vi "log analysis_gps.vi"() -> ()   [LabVIEW 2018] (continued)
0*55731318\n\t", "DUALANTENNAHEADINGA,USB3,0,53.5,FINESTEERING,2107,283868.900,02000000,d426,15824;INSUFFICIENT_OBS,NONE,-1.000000000,0.000000000,0.000000000,0.0,0.000000000,0.000000000,\"631T\",14,3,3,3,04,00,20,00*2bda417b\n\t", "INSPVAXA,USB3,0,47.5,FINESTEERING,2107,283869.400,02000000,471d,15824;INS_ALIGNMENT_COMPLETE,INS_RTKFIXED,37.37070477498,126.72137878954,8.8182,22.3000,-0.3794,-0.2856,0.0387,-0.580248712,0.693765436,214.050059591,0.4343,0.3016,0.5953,0.1139,0.0951,0.0843,0.0965,0.1004,5.1447,0f000001,0*5005ba7a\n\t", "INSPVAXA,USB3,0,47.5,FINESTEERING,2107,283869.900,02000000,471d,15824;INS_ALIGNMENT_COMPLETE,INS_RTKFIXED,37.37070349907,126.72137747347,8.8234,22.3000,-0.3765,-0.2687,0.0325,-0.595922163,0.823980271,213.804726387,0.4343,0.3016,0.5953,0.1139,0.0951,0.0843,0.0965,0.1004,5.1447,0f000001,0*b08e18e5\n\t", "INSPVAXA,USB3,0,48.0,FINESTEERING,2107,283870.400,02000000,471d,15824;INS_ALIGNMENT_COMPLETE,INS_RTKFIXED,37.37070163427,126.72137570159,8.8300,22.3000,-0.3041,-0.2407,0.0180,-0.604642888,0.778196285,214.030795943,0.4340,0.3016,0.5956,0.1141,0.0959,0.0845,0.0966,0.1004,5.1433,0f000001,0*cb822ea1\n\t", "INSPVAXA,USB3,0,48.0,FINESTEERING,2107,283870.900,02000000,471d,15824;INS_ALIGNMENT_COMPLETE,INS_RTKFIXED,37.37069994386,126.72137408130,8.8327,22.3000,-0.4129,-0.3185,0.0299,-0.561714396,1.101086671,213.985768500,0.4340,0.3016,0.5956,0.1141,0.0959,0.0845,0.0966,0.1004,5.1433,0f000001,0*097c1e24\n\t", "INSPVAXA,USB3,0,50.0,FINESTEERING,2107,283871.400,02000000,471d,15824;INS_ALIGNMENT_COMPLETE,INS_RTKFIXED,37.37069831939,126.72137250494,8.8386,22.3000,-0.3879,-0.3050,0.0340,-0.603840717,0.986135442,213.822522610,0.4341,0.3014,0.5961,0.1146,0.0956,0.0852,0.0966,0.1005,5.1404,0f000001,0*99650335\n\t", "INSPVAXA,USB3,0,50.0,FINESTEERING,2107,283871.900,02000000,471d,15824;INS_ALIGNMENT_COMPLETE,INS_RTKFIXED,37.37069663076,126.72137084332,8.8454,22.3000,-0.3570,-0.2814,0.0330,-0.426296070,0.946461964,213.763011209,0.4341,0.3014,0.5961,0.1146,0.0956,0.0852,0.0966,0.1005,5.1404,0f000001,0*8cc6f2c5\n\t", "INSPVAXA,USB3,0,48.5,FINESTEERING,2107,283872.400,02000000,471d,15824;INS_ALIGNMENT_COMPLETE,INS_RTKFIXED,37.37069491831,126.72136922755,8.8525,22.3000,-0.3761,-0.2771,0.0323,-0.638578544,0.908546721,213.728365329,0.4343,0.3024,0.5968,0.1148,0.0958,0.0857,0.0966,0.1006,5.1403,0f000001,0*b6cc0c4e\n\t", "INSPVAXA,USB3,0,48.5,FINESTEERING,2107,283872.900,02000000,471d,15824;INS_ALIGNMENT_COMPLETE,INS_RTKFIXED,37.37069321684,126.72136760945,8.8593,22.3000,-0.3790,-0.2963,0.0419,-0.436104629,0.871418994,213.562317886,0.4343,0.3024,0.5968,0.1148,0.0958,0.0857,0.0966,0.1006,5.1403,0f000001,0*c4a88a6a\n\t", "INSPVAXA,USB3,0,49.5,FINESTEERING,2107,283873.400,02008000,471d,15824;INS_ALIGNMENT_COMPLETE,INS_RTKFIXED,37.37069152716,126.72136602353,8.8633,22.3000,-0.3871,-0.2959,0.0071,-0.372350545,0.744743761,213.502289859,0.4348,0.3034,0.5975,0.1151,0.0961,0.0863,0.0967,0.1006,5.1413,0f000001,0*db4d8b18\n\t", "INSPVAXA,USB3,0,49.5,FINESTEERING,2107,283873.900,02008000,471d,15824;INS_ALIGNMENT_COMPLETE,INS_RTKFIXED,37.37068980188,126.72136442451,8.8669,22.3000,-0.3821,-0.2876,0.0223,-0.542252908,0.493927279,213.372683943,0.4348,0.3034,0.5975,0.1151,0.0961,0.0863,0.0967,0.1006,5.1413,0f000001,0*34acffbe\n\t", "INSPVAXA,USB3,0,52.5,FINESTEERING,2107,283874.400,02008000,471d,15824;INS_ALIGNMENT_COMPLETE,INS_RTKFIXED,37.37068808694,126.72136282059,8.8713,22.3000,-0.3710,-0.2644,0.0357,-0.579423021,0.489216985,213.355766858,0.4351,0.3041,0.5984,0.1155,0.0964,0.0870,0.0968,0.1007,5.1427,0f000001,0*1b568777\n\t", "DUALANTENNAHEADINGA,USB3,0,52.5,FINESTEERING,2107,283874.900,02008000,d426,15824;INSUFFICIENT_OBS,NONE,-1.000000000,0.000000000,0.000000000,0.0,0.000000000,0.000000000,\"631T\",11,3,3,3,04,00,20,00*2cd613df\n\t", "INSPVAXA,USB3,0,49.5,FINESTEERING,2107,283875.400,02008000,471d,15824;INS_ALIGNMENT_COMPLETE,INS_RTKFIXED,37.37068468930,126.72135963115,8.8825,22.3000,-0.3622,-0.2842,0.0299,-0.576500581,0.429092334,213.280984070,0.4354,0.3044,0.5994,0.1156,0.0965,0.0875,0.0969,0.1007,5.1441,0f000001,0*e8de9d75\n\t", "INSPVAXA,USB3,0,49.5,FINESTEERING,2107,283875.900,02008000,471d,15824;INS_ALIGNMENT_COMPLETE,INS_RTKFIXED,37.37068297802,126.72135803904,8.8854,22.3000,-0.3707,-0.2810,0.0365,-0.547997166,0.698496112,213.263606551,0.4354,0.3044,0.5994,0.1156,0.0965,0.0875,0.0969,0.1007,5.1441,0f000001,0*65e2a656\n\t", "INSPVAXA,USB3,0,44.0,FINESTEERING,2107,283876.400,02008000,471d,15824;INS_ALIGNMENT_COMPLETE,INS_RTKFIXED,37.37068125444,126.72135642974,8.8888,22.3000,-0.3786,-0.2878,0.0233,-0.531966030,0.387673420,213.289464944,0.4359,0.3047,0.6005,0.1161,0.0970,0.0885,0.0969,0.1008,5.1456,0f000001,0*b4409e90\n\t", "INSPVAXA,USB3,0,44.0,FINESTEERING,2107,283876.900,02008000,471d,15824;INS_ALIGNMENT_COMPLETE,INS_RTKFIXED,37.37067957761,126.72135484740,8.8937,22.3000,-0.4026,-0.3012,0.0273,-0.420783044,0.494040879,213.316912941,0.4359,0.3047,0.6005,0.1161,0.0970,0.0885,0.0969,0.1008,5.1456,0f000001,0*00e3c1db\n\t", "DUALANTENNAHEADINGA,USB3,0,43.5,FINESTEERING,2107,283877.400,02000000,d426,15824;INSUFFICIENT_OBS,NONE,-1.000000000,0.000000000,0.000000000,0.0,0.000000000,0.000000000,\"631T\",12,3,3,3,04,00,20,00*231fd75a\n\t", "INSPVAXA,USB3,0,43.5,FINESTEERING,2107,283877.900,02000000,471d,15824;INS_ALIGNMENT_COMPLETE,INS_RTKFIXED,37.37067617157,126.72135158509,8.9007,22.3000,-0.3585,-0.2879,0.0250,-0.387485023,0.488203983,213.381189141,0.4358,0.3051,0.6016,0.1150,0.0957,0.0873,0.0971,0.1009,5.1472,0f000001,0*c9483ecc\n\t", "DUALANTENNAHEADINGA,USB3,0,49.5,FINESTEERING,2107,283878.400,02000000,d426,15824;INSUFFICIENT_OBS,NONE,-1.000000000,0.000000000,0.000000000,0.0,0.000000000,0.000000000,\"631T\",9,3,3,3,04,00,20,00*27e46637\n\t", "INSPVAXA,USB3,0,49.5,FINESTEERING,2107,283878.900,02000000,471d,15824;INS_ALIGNMENT_COMPLETE,INS_RTKFIXED,37.37067289269,126.72134842166,8.9107,22.3000,-0.2321,-0.2053,0.0305,-0.361897679,0.347183543,213.363814143,0.4356,0.3048,0.6022,0.1141,0.0948,0.0861,0.0972,0.1010,5.1487,0f000001,0*7c1228c2\n\t", "INSPVAXA,USB3,0,50.0,FINESTEERING,2107,283879.400,02000000,471d,15824;INS_ALIGNMENT_COMPLETE,INS_RTKFIXED,37.37067136914,126.72134696073,8.9138,22.3000,-0.4356,-0.3421,0.0457,-0.368595541,0.477690460,213.236251513,0.4352,0.3048,0.6024,0.1137,0.0954,0.0849,0.0973,0.1011,5.1500,0f000001,0*de91db37\n\t", "DUALANTENNAHEADINGA,USB3,0,50.0,FINESTEERING,2107,283879.900,02000000,d426,15824;INSUFFICIENT_OBS,NONE,-1.000000000,0.000000000,0.000000000,0.0,0.000000000,0.000000000,\"631T\",11,3,3,3,04,00,20,00*7e5de74c\n\t", "INSPVAXA,USB3,0,53.0,FINESTEERING,2107,283880.400,02000000,471d,15824;INS_ALIGNMENT_COMPLETE,INS_RTKFIXED,37.37066797060,126.72134375029,8.9215,22.3000,-0.3538,-0.2783,0.0388,-0.597615608,0.513014169,213.355161065,0.4357,0.3062,0.6023,0.1133,0.0940,0.0839,0.0973,0.1012,5.1494,0f000001,0*cddeff4e\n\t", "INSPVAXA,USB3,0,53.0,FINESTEERING,2107,283880.900,02000000,471d,15824;INS_ALIGNMENT_COMPLETE,INS_RTKFIXED,37.37066635165,126.72134221442,8.9278,22.3000,-0.3658,-0.2852,0.0396,-0.626245150,0.597396810,213.371902809,0.4357,0.3062,0.6023,0.1133,0.0940,0.0839,0.0973,0.1012,5.1494,0f000001,0*bdd5d949\n\t", "DUALANTENNAHEADINGA,USB3,0,50.5,FINESTEERING,2107,283881.400,02000000,d426,15824;INSUFFICIENT_OBS,NONE,-1.000000000,0.000000000,0.000000000,0.0,0.000000000,0.000000000,\"631T\",11,3,3,3,04,00,20,00*4d958a84\n\t", "INSPVAXA,USB3,0,50.5,FINESTEERING,2107,283881.900,02000000,471d,15824;INS_ALIGNMENT_COMPLETE,INS_RTKFIXED,37.37066299197,126.72133897955,8.9361,22.3000,-0.3474,-0.2868,0.0393,-0.593672744,0.610910921,213.511371032,0.4358,0.3048,0.6020,0.1139,0.0948,0.0841,0.0973,0.1012,5.1504,0f000001,0*060d8030\n\t", "DUALANTENNAHEADINGA,USB3,0,51.5,FINESTEERING,2107,283882.400,02000000,d426,15824;INSUFFICIENT_OBS,NONE,-1.000000000,0.000000000,0.000000000,0.0,0.000000000,0.000000000,\"631T\",12,3,3,3,04,00,20,00*3cefd7e2\n\t", "INSPVAXA,USB3,0,51.5,FINESTEERING,2107,283882.900,02000000,471d,15824;INS_ALIGNMENT_COMPLETE,INS_RTKFIXED,37.37065963052,126.72133572900,8.9416,22.3000,-0.3499,-0.2875,0.0236,-0.546470396,0.861326947,213.517075808,0.4357,0.3040,0.6014,0.1142,0.0952,0.0840,0.0973,0.1012,5.1519,0f000001,0*24ce4552\n\t", "INSPVAXA,USB3,0,52.0,FINESTEERING,2107,283883.400,02000000,471d,15824;INS_ALIGNMENT_COMPLETE,INS_RTKFIXED,37.37065796164,126.72133411405,8.9451,22.3000,-0.3685,-0.2983,0.0398,-0.521036438,0.724479041,213.604247881,0.4353,0.3043,0.6007,0.1142,0.0953,0.0836,0.0972,0.1012,5.1533,0f000001,0*63d3ff51\n\t", "DUALANTENNAHEADINGA,USB3,0,52.0,FINESTEERING,2107,283883.900,02000000,d426,15824;INSUFFICIENT_OBS,NONE,-1.000000000,0.000000000,0.000000000,0.0,0.000000000,0.000000000,\"631T\",10,3,3,3,04,00,20,00*65cb768f\n\t", "DUALANTENNAHEADINGA,USB3,0,49.5,FINESTEERING,2107,283884.400,02000000,d426,15824;INSUFFICIENT_OBS,NONE,-1.000000000,0.000000000,0.000000000,0.0,0.000000000,0.000000000,\"631T\",9,3,3,3,04,00,20,00*1d3e0ccf\n\t", "DUALANTENNAHEADINGA,USB3,0,49.5,FINESTEERING,2107,283884.900,02000000,d426,15824;INSUFFICIENT_OBS,NONE,-1.000000000,0.000000000,0.000000000,0.0,0.000000000,0.000000000,\"631T\",10,3,3,3,04,00,20,00*031e6964\n\t", "INSPVAXA,USB3,0,51.5,FINESTEERING,2107,283885.400,02000000,471d,15824;INS_ALIGNMENT_COMPLETE,INS_RTKFIXED,37.37065120654,126.72132762399,8.9567,22.3000,-0.3599,-0.3036,0.0416,-0.421250384,0.704031349,213.500996788,0.4347,0.3046,0.5988,0.1136,0.0944,0.0821,0.0969,0.1010,5.1559,0f000001,0*f6e8d8e3\n\t", "DUALANTENNAHEADINGA,USB3,0,51.5,FINESTEERING,2107,283885.900,02000000,d426,15824;INSUFFICIENT_OBS,NONE,-1.000000000,0.000000000,0.000000000,0.0,0.000000000,0.000000000,\"631T\",9,3,3,3,04,00,20,00*45f2a281\n\t", "DUALANTENNAHEADINGA,USB3,0,53.0,FINESTEERING,2107,283886.400,02000000,d426,15824;INSUFFICIENT_OBS,NONE,-1.000000000,0.000000000,0.000000000,0.0,0.000000000,0.000000000,\"631T\",9,3,3,3,04,00,20,00*f304b34d\n\t", "DUALANTENNAHEADINGA,USB3,0,53.0,FINESTEERING,2107,283886.900,02000000,d426,15824;INSUFFICIENT_OBS,NONE,-1.000000000,0.000000000,0.000000000,0.0,0.000000000,0.000000000,\"631T\",9,3,3,3,04,00,20,00*6aeedf3b\n\t", "DUALANTENNAHEADINGA,USB3,0,53.0,FINESTEERING,2107,283887.400,02000000,d426,15824;INSUFFICIENT_OBS,NONE,-1.000000000,0.000000000,0.000000000,0.0,0.000000000,0.000000000,\"631T\",9,3,3,3,04,00,20,00*f6e48158\n\t", "DUALANTENNAHEADINGA,USB3,0,53.0,FINESTEERING,2107,283887.900,02000000,d426,15824;INSUFFICIENT_OBS,NONE,-1.000000000,0.000000000,0.000000000,0.0,0.000000000,0.000000000,\"631T\",9,3,3,3,04,00,20,00*6f0eed2e\n\t", "DUALANTENNAHEADINGA,USB3,0,52.5,FINESTEERING,2107,283888.400,02000000,d426,15824;INSUFFICIENT_OBS,NONE,-1.000000000,0.000000000,0.000000000,0.0,0.000000000,0.000000000,\"631T\",10,3,3,3,04,00,20,00*e7048907\n\t", "DUALANTENNAHEADINGA,USB3,0,52.5,FINESTEERING,2107,283888.900,02000000,d426,15824;INSUFFICIENT_OBS,NONE,-1.000000000,0.000000000,0.000000000,0.0,0.000000000,0.000000000,\"631T\",10,3,3,3,04,00,20,00*5efbb762\n\t", "DUALANTENNAHEADINGA,USB3,0,46.0,FINESTEERING,2107,283889.400,02000000,d426,15824;INSUFFICIENT_OBS,NONE,-1.000000000,0.000000000,0.000000000,0.0,0.000000000,0.000000000,\"631T\",11,3,3,3,04,00,20,00*93f994bc\n\t", "DUALANTENNAHEADINGA,USB3,0,46.0,FINESTEERING,2107,283889.900,02000000,d426,15824;INSUFFICIENT_OBS,NONE,-1.000000000,0.000000000,0.000000000,0.0,0.000000000,0.000000000,\"631T\",11,3,3,3,04,00,20,00*2a06aad9\n\t", "DUALANTENNAHEADINGA,USB3,0,49.5,FINESTEERING,2107,283890.400,02000000,d426,15824;INSUFFICIENT_OBS,NONE,-1.000000000,0.000000000,0.000000000,0.0,0.000000000,0.000000000,\"631T\",11,3,3,3,04,00,20,00*fe707008\n\t", "DUALANTENNAHEADINGA,USB3,0,49.5,FINESTEERING,2107,283890.900,02000000,d426,15824;INSUFFICIENT_OBS,NONE,-1.000000000,0.000000000,0.000000000,0.0,0.000000000,0.000000000,\"631T\",11,3,3,3,04,00,20,00*478f4e6d\n\t", "DUALANTENNAHEADINGA,USB3,0,50.5,FINESTEERING,2107,283891.400,02000000,d426,15824;INSUFFICIENT_OBS,NONE,-1.000000000,0.000000000,0.000000000,0.0,0.000000000,0.000000000,\"631T\",12,3,3,3,04,00,20,00*11a1be59\n\t", "DUALANTENNAHEADINGA,USB3,0,50.5,FINESTEERING,2107,283891.900,02000000,d426,15824;INSUFFICIENT_OBS,NONE,-1.000000000,0.000000000,0.000000000,0.0,0.000000000,0.000000000,\"631T\",11,3,3,3,04,00,20,00*0b080695\n\t", "DUALANTENNAHEADINGA,USB3,0,51.0,FINESTEERING,2107,283892.400,02000000,d426,15824;INSUFFICIENT_OBS,NONE,-1.000000000,0.000000000,0.000000000,0.0,0.000000000,0.000000000,\"631T\",12,3,3,3,04,00,20,00*96f7835a\n\t", "DUALANTENNAHEADINGA,USB3,0,51.0,FINESTEERING,2107,283892.900,02000000,d426,15824;INSUFFICIENT_OBS,NONE,-1.000000000,0.000000000,0.000000000,0.0,0.000000000,0.000000000,\"631T\",11,3,3,3,04,00,20,00*8c5e3b96\n\t", "DUALANTENNAHEADINGA,USB3,0,50.5,FINESTEERING,2107,283893.400,02000000,d426,15824;INSUFFICIENT_OBS,NONE,-1.000000000,0.000000000,0.000000000,0.0,0.000000000,0.000000000,\"631T\",12,3,3,3,04,00,20,00*ca11b7eb\n\t", "INSPVAXA,USB3,0,50.5,FINESTEERING,2107,283893.900,02000000,471d,15824;INS_ALIGNMENT_COMPLETE,INS_RTKFIXED,37.37062209490,126.72130052647,9.0192,22.3000,-0.3742,-0.3207,0.0346,-0.662095727,0.862366850,212.722532448,0.4356,0.3043,0.5955,0.1140,0.0944,0.0837,0.0963,0.1003,5.1649,0f000001,0*3a5d3b07\n\t", "DUALANTENNAHEADINGA,USB3,0,51.0,FINESTEERING,2107,283894.400,02008000,d426,15824;INSUFFICIENT_OBS,NONE,-1.000000000,0.000000000,0.000000000,0.0,0.000000000,0.000000000,\"631T\",13,3,3,3,04,00,20,00*e0279b34\n\t", "DUALANTENNAHEADINGA,USB3,0,51.0,FINESTEERING,2107,283894.900,02008000,d426,15824;INSUFFICIENT_OBS,NONE,-1.000000000,0.000000000,0.000000000,0.0,0.000000000,0.000000000,\"631T\",14,3,3,3,04,00,20,00*13e62e1a\n\t", "DUALANTENNAHEADINGA,USB3,0,51.0,FINESTEERING,2107,283895.400,02008000,d426,15824;INSUFFICIENT_OBS,NONE,-1.000000000,0.000000000,0.000000000,0.0,0.000000000,0.000000000,\"631T\",12,3,3,3,04,00,20,00*5a1d1fb5\n\t", "DUALANTENNAHEADINGA,USB3,0,51.0,FINESTEERING,2107,283895.900,02008000,d426,15824;INSUFFICIENT_OBS,NONE,-1.000000000,0.000000000,0.000000000,0.0,0.000000000,0.000000000,\"631T\",12,3,3,3,04,00,20,00*e3e221d0\n\t", "DUALANTENNAHEADINGA,USB3,0,51.0,FINESTEERING,2107,283896.400,02008000,d426,15824;INSUFFICIENT_OBS,NONE,-1.000000000,0.000000000,0.000000000,0.0,0.000000000,0.000000000,\"631T\",10,3,3,3,04,00,20,00*98c1142f\n\t", "DUALANTENNAHEADINGA,USB3,0,51.0,FINESTEERING,2107,283896.900,02008000,d426,15824;INSUFFICIENT_OBS,NONE,-1.000000000,0.000000000,0.000000000,0.0,0.000000000,0.000000000,\"631T\",10,3,3,3,04,00,20,00*213e2a4a\n\t", "DUALANTENNAHEADINGA,USB3,0,51.5,FINESTEERING,2107,283897.400,02008000,d426,15824;INSUFFICIENT_OBS,NONE,-1.000000000,0.000000000,0.000000000,0.0,0.000000000,0.000000000,\"631T\",10,3,3,3,04,00,20,00*a063f63a\n\t", "DUALANTENNAHEADINGA,USB3,0,51.5,FINESTEERING,2107,283897.900,02008000,d426,15824;INSUFFICIENT_OBS,NONE,-1.000000000,0.000000000,0.000000000,0.0,0.000000000,0.000000000,\"631T\",10,3,3,3,04,00,20,00*199cc85f\n\t", "DUALANTENNAHEADINGA,USB3,0,52.5,FINESTEERING,2107,283898.400,02008000,d426,15824;INSUFFICIENT_OBS,NONE,-1.000000000,0.000000000,0.000000000,0.0,0.000000000,0.000000000,\"631T\",11,3,3,3,04,00,20,00*d9173f8a\n\t", "DUALANTENNAHEADINGA,USB3,0,52.5,FINESTEERING,2107,283898.900,02008000,d426,15824;INSUFFICIENT_OBS,NONE,-1.000000000,0.000000000,0.000000000,0.0,0.000000000,0.000000000,\"631T\",13,3,3,3,04,00,20,00*145c071e\n\t", "DUALANTENNAHEADINGA,USB3,0,50.5,FINESTEERING,2107,283899.400,02000000,d426,15824;INSUFFICIENT_OBS,NONE,-1.000000000,0.000000000,0.000000000,0.0,0.000000000,0.000000000,\"631T\",15,3,3,3,04,00,20,00*83bd1f58\n\t", "DUALANTENNAHEADINGA,USB3,0,50.5,FINESTEERING,2107,283899.900,02000000,d426,15824;INSUFFICIENT_OBS,NONE,-1.000000000,0.000000000,0.000000000,0.0,0.000000000,0.000000000,\"631T\",11,3,3,3,04,00,20,00*d32a2cdf\n\t", "DUALANTENNAHEADINGA,USB3,0,50.0,FINESTEERING,2107,283900.400,02000000,d426,15824;INSUFFICIENT_OBS,NONE,-1.000000000,0.000000000,0.000000000,0.0,0.000000000,0.000000000,\"631T\",9,3,3,3,04,00,20,00*b9862b26\n\t", "DUALANTENNAHEADINGA,USB3,0,50.0,FINESTEERING,2107,283900.900,02000000,d426,15824;INSUFFICIENT_OBS,NONE,-1.000000000,0.000000000,0.000000000,0.0,0.000000000,0.000000000,\"631T\",9,3,3,3,04,00,20,00*206c4750\n\t", "DUALANTENNAHEADINGA,USB3,0,50.0,FINESTEERING,2107,283901.400,02008000,d426,15824;INSUFFICIENT_OBS,NONE,-1.000000000,0.000000000,0.000000000,0.0,0.000000000,0.000000000,\"631T\",9,3,3,3,04,00,20,00*432dfdec\n\t", "DUALANTENNAHEADINGA,USB3,0,50.0,FINESTEERING,2107,283902.400,02008000,d426,15824;INSUFFICIENT_OBS,NONE,-1.000000000,0.000000000,0.000000000,0.0,0.000000000,0.000000000,\"631T\",11,3,3,3,04,00,20,00*7952b8b1\n\t", "DUALANTENNAHEADINGA,USB3,0,50.0,FINESTEERING,2107,283902.900,02008000,d426,15824;INSUFFICIENT_OBS,NONE,-1.000000000,0.000000000,0.000000000,0.0,0.000000000,0.000000000,\"631T\",10,3,3,3,04,00,20,00*174f068c\n\t", "INSPVAXA,USB3,0,49.0,FINESTEERING,2107,283903.450,02008000,471d,15824;INS_ALIGNMENT_COMPLETE,INS_RTKFIXED,37.37058884071,126.72127040415,9.0705,22.3000,-0.3807,-0.3020,0.0207,-0.679787264,0.064920800,213.254026909,0.4334,0.3029,0.5969,0.1133,0.0944,0.0822,0.0966,0.1006,5.1769,0f000001,0*71c893b5\n\t", "DUALANTENNAHEADINGA,USB3,0,48.5,FINESTEERING,2107,283904.400,02008000,d426,15824;INSUFFICIENT_OBS,NONE,-1.000000000,0.000000000,0.000000000,0.0,0.000000000,0.000000000,\"631T\",11,3,3,3,04,00,20,00*de92d86f\n\t", "INSPVAXA,USB3,0,48.5,FINESTEERING,2107,283904.950,02008000,471d,15824;INS_ALIGNMENT_COMPLETE,INS_RTKFIXED,37.37058369457,126.72126562815,9.0689,22.3000,-0.3526,-0.2989,0.0165,-0.611939006,0.199763029,213.494948606,0.4333,0.3029,0.5964,0.1131,0.0941,0.0816,0.0965,0.1006,5.1782,0f000001,0*4f2b9d43\n\t", "DUALANTENNAHEADINGA,USB3,0,51.0,FINESTEERING,2107,283905.400,02000000,d426,15824;INSUFFICIENT_OBS,NONE,-1.000000000,0.000000000,0.000000000,0.0,0.000000000,0.000000000,\"631T\",11,3,3,3,04,00,20,00*d1fcf2fa\n\t", "INSPVAXA,USB3,0,51.0,FINESTEERING,2107,283905.950,02000000,471d,15824;INS_ALIGNMENT_COMPLETE,INS_RTKFIXED,37.37058025923,126.72126241939,9.0707,22.3000,-0.3812,-0.3080,0.0278,-0.525044361,0.591334106,213.674985050,0.4335,0.3031,0.5959,0.1142,0.0952,0.0829,0.0965,0.1005,5.1795,0f000001,0*069603aa\n\t", "DUALANTENNAHEADINGA,USB3,0,50.0,FINESTEERING,2107,283906.400,02000000,d426,15824;INSUFFICIENT_OBS,NONE,-1.000000000,0.000000000,0.000000000,0.0,0.000000000,0.000000000,\"631T\",11,3,3,3,04,00,20,00*03d02935\n\t", "INSPVAXA,USB3,0,50.0,FINESTEERING,2107,283906.950,02000000,471d,15824;INS_ALIGNMENT_COMPLETE,INS_RTKFIXED,37.37057686520,126.72125915274,9.0748,22.3000,-0.3835,-0.3158,0.0154,-0.714794692,0.316524554,214.061130278,0.4338,0.3036,0.5955,0.1138,0.0946,0.0824,0.0964,0.1005,5.1810,0f000001,0*ecb7aa1d\n\t", "DUALANTENNAHEADINGA,USB3,0,51.0,FINESTEERING,2107,283907.400,02000000,d426,15824;INSUFFICIENT_OBS,NONE,-1.000000000,0.000000000,0.000000000,0.0,0.000000000,0.000000000,\"631T\",12,3,3,3,04,00,20,00*a91a7de1\n\t", "DUALANTENNAHEADINGA,USB3,0,51.0,FINESTEERING,2107,283907.900,02000000,d426,15824;INSUFFICIENT_OBS,NONE,-1.000000000,0.000000000,0.000000000,0.0,0.000000000,0.000000000,\"631T\",11,3,3,3,04,00,20,00*b3b3c52d\n\t", "DUALANTENNAHEADINGA,USB3,0,52.5,FINESTEERING,2107,283908.900,02000000,d426,15824;INSUFFICIENT_OBS,NONE,-1.000000000,0.000000000,0.000000000,0.0,0.000000000,0.000000000,\"631T\",11,3,3,3,04,00,20,00*485f6a09\n\t", "DUALANTENNAHEADINGA,USB3,0,50.5,FINESTEERING,2107,283909.400,02000000,d426,15824;INSUFFICIENT_OBS,NONE,-1.000000000,0.000000000,0.000000000,0.0,0.000000000,0.000000000,\"631T\",12,3,3,3,04,00,20,00*f7a77b54\n\t", "DUALANTENNAHEADINGA,USB3,0,50.5,FINESTEERING,2107,283909.900,02000000,d426,15824;INSUFFICIENT_OBS,NONE,-1.000000000,0.000000000,0.000000000,0.0,0.000000000,0.000000000,\"631T\",13,3,3,3,04,00,20,00*99bac569\n\t", "INSPVAXA,USB3,0,48.0,FINESTEERING,2107,283910.450,02000000,471d,15824;INS_ALIGNMENT_COMPLETE,INS_RTKFIXED,37.37056496909,126.72124764665,9.0863,22.3000,-0.3554,-0.3247,0.0202,-0.305074143,0.317241831,214.523867584,0.4346,0.3048,0.5954,0.1134,0.0941,0.0823,0.0963,0.1003,5.1868,0f000001,0*02f445bc\n\t", "DUALANTENNAHEADINGA,USB3,0,48.0,FINESTEERING,2107,283910.900,02000000,d426,15824;INSUFFICIENT_OBS,NONE,-1.000000000,0.000000000,0.000000000,0.0,0.000000000,0.000000000,\"631T\",12,3,3,3,04,00,20,00*14a1a59f\n\t", "INSPVAXA,USB3,0,49.5,FINESTEERING,2107,283911.450,02000000,471d,15824;INS_ALIGNMENT_COMPLETE,INS_RTKFIXED,37.37056161289,126.72124438523,9.0878,22.3000,-0.3391,-0.2889,0.0305,-0.373763892,0.193972280,214.477350215,0.4341,0.3042,0.5952,0.1138,0.0946,0.0829,0.0963,0.1003,5.1884,0f000001,0*19e64a77\n\t", "DUALANTENNAHEADINGA,USB3,0,51.0,FINESTEERING,2107,283912.400,02000000,d426,15824;INSUFFICIENT_OBS,NONE,-1.000000000,0.000000000,0.000000000,0.0,0.000000000,0.000000000,\"631T\",10,3,3,3,04,00,20,00*2305d898\n\t", "INSPVAXA,USB3,0,51.0,FINESTEERING,2107,283912.950,02000000,471d,15824;INS_ALIGNMENT_COMPLETE,INS_RTKFIXED,37.37055667019,126.72123951954,9.0936,22.3000,-0.3847,-0.3125,0.0281,-0.432078717,0.899277400,214.193265396,0.4336,0.3036,0.5951,0.1137,0.0947,0.0831,0.0963,0.1003,5.1898,0f000001,0*1102a532\n\t", "DUALANTENNAHEADINGA,USB3,0,52.5,FINESTEERING,2107,283913.400,02000000,d426,15824;INSUFFICIENT_OBS,NONE,-1.000000000,0.000000000,0.000000000,0.0,0.000000000,0.000000000,\"631T\",11,3,3,3,04,00,20,00*6088c139\n\t", "DUALANTENNAHEADINGA,USB3,0,52.5,FINESTEERING,2107,283913.900,02000000,d426,15824;INSUFFICIENT_OBS,NONE,-1.000000000,0.000000000,0.000000000,0.0,0.000000000,0.000000000,\"631T\",13,3,3,3,04,00,20,00*adc3f9ad\n\t", "INSPVAXA,USB3,0,48.0,FINESTEERING,2107,283914.450,02000000,471d,15824;INS_ALIGNMENT_COMPLETE,INS_RTKFIXED,37.37055172372,126.72123465908,9.1045,22.3000,-0.3321,-0.3029,0.0193,-0.498508011,0.792000262,213.719525231,0.4335,0.3037,0.5952,0.1132,0.0940,0.0823,0.0963,0.1003,5.1929,0f000001,0*c17a4193\n\t", "INSPVAXA,USB3,0,48.0,FINESTEERING,2107,283914.950,02000000,471d,15824;INS_ALIGNMENT_COMPLETE,INS_RTKFIXED,37.37055006660,126.72123300626,9.1068,22.3000,-0.3507,-0.2983,0.0012,-0.233266820,0.708375211,213.616604793,0.4335,0.3037,0.5952,0.1132,0.0940,0.0823,0.0963,0.1003,5.1929,0f000001,0*8c718c31\n\t", "DUALANTENNAHEADINGA,USB3,0,47.0,FINESTEERING,2107,283915.400,02000000,d426,15824;INSUFFICIENT_OBS,NONE,-1.000000000,0.000000000,0.000000000,0.0,0.000000000,0.000000000,\"631T\",11,3,3,3,04,00,20,00*7daa9230\n\t", "INSPVAXA,USB3,0,47.0,FINESTEERING,2107,283915.950,02000000,471d,15824;INS_ALIGNMENT_COMPLETE,INS_RTKFIXED,37.37054673087,126.72122978879,9.1114,22.3000,-0.3591,-0.2902,0.0351,-0.280063258,0.768282729,213.379617811,0.4334,0.3035,0.5951,0.1128,0.0937,0.0818,0.0963,0.1003,5.1943,0f000001,0*df737fc9\n\t", "INSPVAXA,USB3,0,49.0,FINESTEERING,2107,283916.450,02000000,471d,15824;INS_ALIGNMENT_COMPLETE,INS_RTKFIXED,37.37054503635,126.72122820634,9.1136,22.3000,-0.3595,-0.2800,0.0167,-0.568627617,0.574232692,213.297475739,0.4336,0.3033,0.5948,0.1126,0.0935,0.0813,0.0963,0.1003,5.1956,0f000001,0*cacfced8\n\t", "INSPVAXA,USB3,0,49.0,FINESTEERING,2107,283916.950,02000000,471d,15824;INS_ALIGNMENT_COMPLETE,INS_RTKFIXED,37.37054332182,126.72122657762,9.1146,22.3000,-0.3450,-0.3025,0.0148,-0.530748763,0.232275373,213.084868526,0.4336,0.3033,0.5948,0.1126,0.0935,0.0813,0.0963,0.1003,5.1956,0f000001,0*d44f9e4e\n\t", "INSPVAXA,USB3,0,49.0,FINESTEERING,2107,283917.450,02000000,471d,15824;INS_ALIGNMENT_COMPLETE,INS_RTKFIXED,37.37054163352,126.72122501811,9.1165,22.3000,-0.3554,-0.2975,0.0340,-0.824959720,0.443504930,213.062065508,0.4333,0.3029,0.5945,0.1125,0.0935,0.0809,0.0963,0.1003,5.1969,0f000001,0*c7e22c84\n\t", "DUALANTENNAHEADINGA,USB3,0,50.5,FINESTEERING,2107,283918.400,02000000,d426,15824;INSUFFICIENT_OBS,NONE,-1.000000000,0.000000000,0.000000000,0.0,0.000000000,0.000000000,\"631T\",9,3,3,3,04,00,20,00*849f5ce0\n\t", "INSPVAXA,USB3,0,50.5,FINESTEERING,2107,283918.950,02000000,471d,15824;INS_ALIGNMENT_COMPLETE,INS_RTKFIXED,37.37053657031,126.72122025773,9.1231,22.3000,-0.3626,-0.3082,0.0292,-0.664128587,0.419081296,212.844872537,0.4329,0.3028,0.5939,0.1124,0.0937,0.0805,0.0963,0.1003,5.1982,0f000001,0*4b642c0a\n\t", "INSPVAXA,USB3,0,47.0,FINESTEERING,2107,283919.450,02000000,471d,15824;INS_ALIGNMENT_COMPLETE,INS_RTKFIXED,37.37053487627,126.72121868660,9.1237,22.3000,-0.3564,-0.3030,0.0002,-0.479328708,0.369667523,212.741899400,0.4326,0.3022,0.5934,0.1124,0.0936,0.0802,0.0962,0.1003,5.1992,0f000001,0*77fc8fa5\n\t", "INSPVAXA,USB3,0,47.0,FINESTEERING,2107,283919.950,02000000,471d,15824;INS_ALIGNMENT_COMPLETE,INS_RTKFIXED,37.37053314698,126.72121706257,9.1241,22.3000,-0.3522,-0.3058,0.0197,-0.363383073,0.096459549,212.853457646,0.4326,0.3022,0.5934,0.1124,0.0936,0.0802,0.0962,0.1003,5.1992,0f000001,0*a718023e\n\t", "INSPVAXA,USB3,0,52.0,FINESTEERING,2107,283920.450,02000000,471d,15824;INS_ALIGNMENT_COMPLETE,INS_RTKFIXED,37.37053146524,126.72121553588,9.1258,22.3000,-0.3500,-0.2976,0.0272,-0.521767170,0.221904426,212.799458593,0.4324,0.3020,0.5928,0.1125,0.0936,0.0799,0.0961,0.1002,5.2000,0f000001,0*115d72dc\n\t", "INSPVAXA,USB3,0,48.0,FINESTEERING,2107,283921.450,02000000,471d,15824;INS_ALIGNMENT_COMPLETE,INS_RTKFIXED,37.37052802282,126.72121240001,9.1291,22.3000,-0.3507,-0.3057,0.0251,-0.215783432,0.396063272,212.883809512,0.4322,0.3017,0.5920,0.1125,0.0935,0.0797,0.0960,0.1002,5.2006,0f000001,0*28d97cd1\n\t", "INSPVAXA,USB3,0,48.0,FINESTEERING,2107,283921.950,02000000,471d,15824;INS_ALIGNMENT_COMPLETE,INS_RTKFIXED,37.37052634631,126.72121089774,9.1341,22.3000,-0.3596,-0.2838,0.0323,-0.415372337,0.706980969,212.926580959,0.4322,0.3017,0.5920,0.1125,0.0935,0.0797,0.0960,0.1002,5.2006,0f000001,0*148fe8d6\n\t", "INSPVAXA,USB3,0,43.0,FINESTEERING,2107,283922.450,02000000,471d,15824;INS_ALIGNMENT_COMPLETE,INS_RTKFIXED,37.37052460357,126.72120933072,9.1390,22.3000,-0.3446,-0.3015,0.0137,-0.382873007,0.563010953,212.928415689,0.4322,0.3018,0.5913,0.1124,0.0934,0.0795,0.0959,0.1001,5.2012,0f000001,0*06ecfb60\n\t", "INSPVAXA,USB3,0,43.0,FINESTEERING,2107,283922.950,02000000,471d,15824;INS_ALIGNMENT_COMPLETE,INS_RTKFIXED,37.37052292197,126.72120779195,9.1447,22.3000,-0.3494,-0.2921,0.0334,-0.254339897,0.526441587,212.988420393,0.4322,0.3018,0.5913,0.1124,0.0934,0.0795,0.0959,0.1001,5.2012,0f000001,0*74466e11\n\t", "INSPVAXA,USB3,0,45.5,FINESTEERING,2107,283923.450,02000000,471d,15824;INS_ALIGNMENT_COMPLETE,INS_RTKFIXED,37.37052118554,126.72120621046,9.1491,22.3000,-0.3583,-0.2946,0.0183,-0.080875673,0.518402555,213.021069152,0.4321,0.3020,0.5906,0.1124,0.0934,0.0794,0.0958,0.1001,5.2021,0f000001,0*09f1c4be\n\t", "INSPVAXA,USB3,0,45.5,FINESTEERING,2107,283923.950,02000000,471d,15824;INS_ALIGNMENT_COMPLETE,INS_RTKFIXED,37.37051949937,126.72120468984,9.1523,22.3000,-0.3577,-0.2933,0.0036,-0.207836211,0.548820152,213.042486887,0.4321,0.3020,0.5906,0.1124,0.0934,0.0794,0.0958,0.1001,5.2021,0f000001,0*e62c9616\n\t", "INSPVAXA,USB3,0,50.0,FINESTEERING,2107,283924.450,02000000,471d,15824;INS_ALIGNMENT_COMPLETE,INS_RTKFIXED,37.37051776431,126.72120311911,9.1553,22.3000,-0.3480,-0.2880,0.0361,-0.209670609,0.595606109,213.112162287,0.4321,0.3024,0.5900,0.1124,0.0933,0.0793,0.0957,0.1000,5.2033,0f000001,0*9cc91f60\n\t", "INSPVAXA,USB3,0,50.0,FINESTEERING,2107,283924.950,02000000,471d,15824;INS_ALIGNMENT_COMPLETE,INS_RTKFIXED,37.37051602540,126.72120154897,9.1565,22.3000,-0.3460,-0.2879,0.0300,-0.302016421,0.742841362,213.157571504,0.4321,0.3024,0.5900,0.1124,0.0933,0.0793,0.0957,0.1000,5.2033,0f000001,0*c2c8a9b5\n\t", "INSPVAXA,USB3,0,50.5,FINESTEERING,2107,283925.450,02000000,471d,15824;INS_ALIGNMENT_COMPLETE,INS_RTKFIXED,37.37051431661,126.72119998698,9.1612,22.3000,-0.3602,-0.3017,0.0078,-0.150276510,0.673330770,213.275693569,0.4320,0.3027,0.5895,0.1123,0.0933,0.0792,0.0956,0.1000,5.2048,0f000001,0*406b8736\n\t", "INSPVAXA,USB3,0,50.5,FINESTEERING,2107,283925.950,02000000,471d,15824;INS_ALIGNMENT_COMPLETE,INS_RTKFIXED,37.37051260472,126.72119841122,9.1660,22.3000,-0.3548,-0.3097,0.0154,-0.098276795,0.507978734,213.441186851,0.4320,0.3027,0.5895,0.1123,0.0933,0.0792,0.0956,0.1000,5.2048,0f000001,0*9b14382d\n\t", "DUALANTENNAHEADINGA,USB3,0,48.5,FINESTEERING,2107,283926.400,02000000,d426,15824;INSUFFICIENT_OBS,NONE,-1.000000000,0.000000000,0.000000000,0.0,0.000000000,0.000000000,\"631T\",10,3,3,3,04,00,20,00*e1e7b78d\n\t", "INSPVAXA,USB3,0,48.5,FINESTEERING,2107,283926.950,02000000,471d,15824;INS_ALIGNMENT_COMPLETE,INS_RTKFIXED,37.37050917237,126.72119519528,9.1767,22.3000,-0.3519,-0.3025,0.0208,-0.173094935,0.655730796,213.776498687,0.4320,0.3032,0.5892,0.1131,0.0942,0.0804,0.0956,0.0999,5.2064,0f000001,0*f79ccc8c\n\t", "INSPVAXA,USB3,0,45.5,FINESTEERING,2107,283927.450,02000000,471d,15824;INS_ALIGNMENT_COMPLETE,INS_RTKFIXED,37.37050743516,126.72119359440,9.1795,22.3000,-0.3580,-0.2979,0.0147,-0.110231872,0.525103385,214.016806348,0.4321,0.3036,0.5890,0.1128,0.0938,0.0803,0.0956,0.0999,5.2080,0f000001,0*f1eaf58d\n\t", "INSPVAXA,USB3,0,45.5,FINESTEERING,2107,283927.950,02000000,471d,15824;INS_ALIGNMENT_COMPLETE,INS_RTKFIXED,37.37050571191,126.72119201313,9.1838,22.3000,-0.3640,-0.2912,0.0308,-0.267249738,0.507353767,214.246041295,0.4321,0.3036,0.5890,0.1128,0.0938,0.0803,0.0956,0.0999,5.2080,0f000001,0*5bacc05f\n\t", "INSPVAXA,USB3,0,49.0,FINESTEERING,2107,283928.450,02000000,471d,15824;INS_ALIGNMENT_COMPLETE,INS_RTKFIXED,37.37050398059,126.72119038218,9.1856,22.3000,-0.3631,-0.3028,0.0151,-0.368561001,0.456085807,214.459019955,0.4324,0.3038,0.5890,0.1126,0.0935,0.0802,0.0956,0.0998,5.2095,0f000001,0*73c86a57\n\t", "INSPVAXA,USB3,0,49.0,FINESTEERING,2107,283928.950,02000000,471d,15824;INS_ALIGNMENT_COMPLETE,INS_RTKFIXED,37.37050228349,126.72118877638,9.1897,22.3000,-0.3679,-0.3047,0.0058,-0.525199888,0.456229866,214.593983111,0.4324,0.3038,0.5890,0.1126,0.0935,0.0802,0.0956,0.0998,5.2095,0f000001,0*0c17fda2\n\t", "INSPVAXA,USB3,0,48.0,FINESTEERING,2107,283929.450,02000000,471d,15824;INS_ALIGNMENT_COMPLETE,INS_RTKFIXED,37.37050057739,126.72118712143,9.1936,22.3000,-0.3554,-0.3037,0.0227,-0.396145969,0.312216334,214.731264498,0.4324,0.3037,0.5892,0.1125,0.0933,0.0800,0.0956,0.0998,5.2109,0f000001,0*e8b24b74\n\t", "INSPVAXA,USB3,0,48.0,FINESTEERING,2107,283929.950,02000000,471d,15824;INS_ALIGNMENT_COMPLETE,INS_RTKFIXED,37.37049890881,126.72118550326,9.1969,22.3000,-0.3488,-0.2994,0.0296,-0.491904024,0.536179959,214.904903866,0.4324,0.3037,0.5892,0.1125,0.0933,0.0800,0.0956,0.0998,5.2109,0f000001,0*ad87a7a5\n\t", "INSPVAXA,USB3,0,48.5,FINESTEERING,2107,283930.450,02000000,471d,15824;INS_ALIGNMENT_COMPLETE,INS_RTKFIXED,37.37049721050,126.72118386884,9.1995,22.3000,-0.3636,-0.2994,0.0018,-0.629398853,0.403170896,215.071222614,0.4325,0.3033,0.5894,0.1129,0.0937,0.0807,0.0956,0.0998,5.2121,0f000001,0*cd026204\n\t", "INSPVAXA,USB3,0,48.5,FINESTEERING,2107,283930.950,02000000,471d,15824;INS_ALIGNMENT_COMPLETE,INS_RTKFIXED,37.37049554136,126.72118223903,9.2033,22.3000,-0.3579,-0.3114,0.0267,-0.630465931,0.456383664,215.164754622,0.4325,0.3033,0.5894,0.1129,0.0937,0.0807,0.0956,0.0998,5.2121,0f000001,0*d7b4217a\n\t", "INSPVAXA,USB3,0,51.0,FINESTEERING,2107,283931.450,02000000,471d,15824;INS_ALIGNMENT_COMPLETE,INS_RTKFIXED,37.37049384282,126.72118058399,9.2075,22.3000,-0.3544,-0.2989,0.0161,-0.740038291,0.456521512,215.355756173,0.4326,0.3033,0.5897,0.1135,0.0944,0.0819,0.0956,0.0998,5.2130,0f000001,0*1b20caf7\n\t", "INSPVAXA,USB3,0,51.0,FINESTEERING,2107,283931.950,02000000,471d,15824;INS_ALIGNMENT_COMPLETE,INS_RTKFIXED,37.37049213218,126.72117889345,9.2111,22.3000,-0.3596,-0.3121,0.0183,-0.657813953,0.413680306,215.408958644,0.4326,0.3033,0.5897,0.1135,0.0944,0.0819,0.0956,0.0998,5.2130,0f000001,0*a46484af\n\t", "INSPVAXA,USB3,0,50.0,FINESTEERING,2107,283932.450,02000000,471d,15824;INS_ALIGNMENT_COMPLETE,INS_RTKFIXED,37.37049046733,126.72117722659,9.2158,22.3000,-0.3473,-0.3092,0.0349,-0.590608670,0.319388706,215.361013781,0.4329,0.3036,0.5903,0.1143,0.0953,0.0834,0.0957,0.0998,5.2135,0f000001,0*5573a11c\n\t", "INSPVAXA,USB3,0,50.0,FINESTEERING,2107,283932.950,02000000,471d,15824;INS_ALIGNMENT_COMPLETE,INS_RTKFIXED,37.37048877805,126.72117553421,9.2224,22.3000,-0.3576,-0.3071,0.0334,-0.545773763,0.550162659,215.419033819,0.4329,0.3036,0.5903,0.1143,0.0953,0.0834,0.0957,0.0998,5.2135,0f000001,0*06d0156c\n\t", "INSPVAXA,USB3,0,46.5,FINESTEERING,2107,283933.450,02000000,471d,15824;INS_ALIGNMENT_COMPLETE,INS_RTKFIXED,37.37048709327,126.72117385484,9.2273,22.3000,-0.3583,-0.3032,0.0201,-0.584226709,0.709789470,215.528367136,0.4335,0.3040,0.5913,0.1137,0.0945,0.0830,0.0957,0.0998,5.2139,0f000001,0*ba7d8e29\n\t", "INSPVAXA,USB3,0,46.5,FINESTEERING,2107,283933.950,02000000,471d,15824;INS_ALIGNMENT_COMPLETE,INS_RTKFIXED,37.37048540421,126.72117215519,9.2325,22.3000,-0.3686,-0.3092,0.0093,-0.663238373,0.676190653,215.463359493,0.4335,0.3040,0.5913,0.1137,0.0945,0.0830,0.0957,0.0998,5.2139,0f000001,0*5a7d9a35\n\t", "INSPVAXA,USB3,0,51.5,FINESTEERING,2107,283934.450,02000000,471d,15824;INS_ALIGNMENT_COMPLETE,INS_RTKFIXED,37.37048375352,126.72117048246,9.2375,22.3000,-0.3734,-0.3205,0.0340,-0.435969106,0.945574003,215.391049185,0.4334,0.3041,0.5920,0.1131,0.0939,0.0826,0.0958,0.0998,5.2143,0f000001,0*bcbd8a70\n\t", "INSPVAXA,USB3,0,51.5,FINESTEERING,2107,283934.950,02000000,471d,15824;INS_ALIGNMENT_COMPLETE,INS_RTKFIXED,37.37048205847,126.72116880230,9.2433,22.3000,-0.3752,-0.3030,0.0191,-0.551123480,0.797684003,215.136467002,0.4334,0.3041,0.5920,0.1131,0.0939,0.0826,0.0958,0.0998,5.2143,0f000001,0*2d6be551\n\t", "INSPVAXA,USB3,0,49.0,FINESTEERING,2107,283935.950,02000000,471d,15824;INS_ALIGNMENT_COMPLETE,INS_RTKFIXED,37.37047866137,126.72116545098,9.2537,22.3000,-0.3697,-0.3129,0.0257,-0.409292319,0.632531125,214.781702011,0.4334,0.3038,0.5927,0.1127,0.0935,0.0821,0.0959,0.0999,5.2145,0f000001,0*763cf472\n\t", "INSPVAXA,USB3,0,48.0,FINESTEERING,2107,283936.450,02000000,471d,15824;INS_ALIGNMENT_COMPLETE,INS_RTKFIXED,37.37047695933,126.72116379842,9.2575,22.3000,-0.3601,-0.2905,0.0223,-0.510166928,0.275357051,214.549267942,0.4332,0.3032,0.5933,0.1122,0.0932,0.0817,0.0960,0.0999,5.2143,0f000001,0*907ae007\n\t", "INSPVAXA,USB3,0,48.0,FINESTEERING,2107,283936.950,02000000,471d,15824;INS_ALIGNMENT_COMPLETE,INS_RTKFIXED,37.37047527853,126.72116215716,9.2617,22.3000,-0.3613,-0.3073,0.0319,-0.493749348,0.435637715,214.244212344,0.4332,0.3032,0.5933,0.1122,0.0932,0.0817,0.0960,0.0999,5.2143,0f000001,0*77c5d1d8\n\t", "INSPVAXA,USB3,0,48.5,FINESTEERING,2107,283937.950,02000000,471d,15824;INS_ALIGNMENT_COMPLETE,INS_RTKFIXED,37.37047189710,126.72115890646,9.2688,22.3000,-0.3586,-0.2934,0.0244,-0.533486904,0.671561834,213.833990455,0.4328,0.3028,0.5937,0.1126,0.0939,0.0822,0.0961,0.1000,5.2146,0f000001,0*9215f66d\n\t", "INSPVAXA,USB3,0,52.0,FINESTEERING,2107,283938.450,02000000,471d,15824;INS_ALIGNMENT_COMPLETE,INS_RTKFIXED,37.37047020437,126.72115727420,9.2725,22.3000,-0.3547,-0.3143,0.0241,-0.356445317,0.659835202,213.629028548,0.4325,0.3026,0.5940,0.1125,0.0937,0.0818,0.0961,0.1000,5.2151,0f000001,0*9a205bce\n\t", "INSPVAXA,USB3,0,52.0,FINESTEERING,2107,283938.950,02000000,471d,15824;INS_ALIGNMENT_COMPLETE,INS_RTKFIXED,37.37046851551,126.72115567512,9.2776,22.3000,-0.3685,-0.3042,0.0189,-0.419579821,0.629946557,213.500724202,0.4325,0.3026,0.5940,0.1125,0.0937,0.0818,0.0961,0.1000,5.2151,0f000001,0*4752d92c\n\t", "INSPVAXA,USB3,0,49.5,FINESTEERING,2107,283939.950,02000000,471d,15824;INS_ALIGNMENT_COMPLETE,INS_RTKFIXED,37.37046510443,126.72115247371,9.2872,22.3000,-0.3830,-0.2927,0.0256,-0.146641459,0.857904302,213.119748571,0.4322,0.3028,0.5939,0.1123,0.0936,0.0813,0.0961,0.1000,5.2160,0f000001,0*783a43e7\n\t", "INSPVAXA,USB3,0,46.5,FINESTEERING,2107,283941.950,02000000,471d,15824;INS_ALIGNMENT_COMPLETE,INS_RTKFIXED,37.37045819174,126.72114613372,9.3070,22.3000,-0.3933,-0.3167,0.0134,-0.360308060,0.744674803,212.733059130,0.4319,0.3027,0.5939,0.1126,0.0939,0.0813,0.0961,0.1000,5.2180,0f000001,0*c8f7eb70\n\t", "INSPVAXA,USB3,0,51.5,FINESTEERING,2107,283944.450,02000000,471d,15824;INS_ALIGNMENT_COMPLETE,INS_RTKFIXED,37.37044958989,126.72113821345,9.3358,22.3000,-0.3641,-0.3051,0.0226,-0.383976023,0.466369784,212.614223269,0.4320,0.3035,0.5933,0.1137,0.0952,0.0823,0.0960,0.1000,5.2226,0f000001,0*0b47cfbf\n\t", "INSPVAXA,USB3,0,51.0,FINESTEERING,2107,283945.950,02000000,471d,15824;INS_ALIGNMENT_COMPLETE,INS_RTKFIXED,37.37044449644,126.72113345903,9.3530,22.3000,-0.3492,-0.2810,0.0259,-0.492056173,0.868162173,212.637209572,0.4322,0.3030,0.5933,0.1133,0.0945,0.0819,0.0959,0.1000,5.2239,0f000001,0*fbf44ee4\n\t", "INSPVAXA,USB3,0,50.5,FINESTEERING,2107,283947.950,02000000,471d,15824;INS_ALIGNMENT_COMPLETE,INS_RTKFIXED,37.37043763245,126.72112720109,9.3747,22.3000,-0.3517,-0.2756,0.0362,-0.981277004,0.835950889,212.295904790,0.4324,0.3035,0.5933,0.1126,0.0937,0.0812,0.0959,0.0999,5.2264,0f000001,0*ec5c30da\n\t", "INSPVAXA,USB3,0,51.0,FINESTEERING,2107,283948.450,02000000,471d,15824;INS_ALIGNMENT_COMPLETE,INS_RTKFIXED,37.37043588029,126.72112562917,9.3803,22.3000,-0.3710,-0.2973,0.0467,-0.738282510,0.795123885,212.189518726,0.4321,0.3032,0.5932,0.1125,0.0934,0.0808,0.0959,0.0999,5.2279,0f000001,0*ed2f12b7\n\t", "INSPVAXA,USB3,0,50.5,FINESTEERING,2107,283953.450,02008000,471d,15824;INS_ALIGNMENT_COMPLETE,INS_RTKFIXED,37.37041847684,126.72111045346,9.4216,22.3000,-0.3714,-0.2867,0.0304,-1.344882424,0.718506073,211.705510005,0.4322,0.3022,0.5921,0.1132,0.0948,0.0813,0.0958,0.0998,5.2323,0f000001,0*748620fd\n\t", "INSPVAXA,USB3,0,48.5,FINESTEERING,2107,283975.500,02000000,471d,15824;INS_ALIGNMENT_COMPLETE,INS_RTKFIXED,37.37034183103,126.72104365598,9.5499,22.3000,-0.3648,-0.2725,0.0197,-1.244402765,0.202153747,211.898676033,0.4326,0.3045,0.5916,0.1133,0.0944,0.0814,0.0956,0.0997,5.2502,0f000001,0*746e4bd4\n\t", "INSPVAXA,USB3,0,50.5,FINESTEERING,2107,283979.000,02000000,471d,15824;INS_ALIGNMENT_COMPLETE,INS_RTKFIXED,37.37032960177,126.72103274756,9.5709,22.3000,-0.3611,-0.2914,0.0231,-1.123681308,0.223311003,213.340300492,0.4324,0.3037,0.5929,0.1134,0.0946,0.0828,0.0957,0.0996,5.2509,0f000001,0*020bc469\n\t", "INSPVAXA,USB3,0,51.5,FINESTEERING,2107,283980.000,02000000,471d,15824;INS_ALIGNMENT_COMPLETE,INS_RTKFIXED,37.37032615968,126.72102953721,9.5775,22.3000,-0.3586,-0.2940,0.0139,-1.097113995,0.335693778,213.663017986,0.4326,0.3036,0.5938,0.1129,0.0941,0.0824,0.0958,0.0997,5.2514,0f000001,0*6db47364\n\t", "INSPVAXA,USB3,0,49.5,FINESTEERING,2107,283981.500,02008000,471d,15824;INS_ALIGNMENT_COMPLETE,INS_RTKFIXED,37.37032104015,126.72102467256,9.5879,22.3000,-0.3441,-0.2878,0.0186,-1.054014794,0.825950094,214.092959020,0.4321,0.3029,0.5950,0.1124,0.0936,0.0820,0.0959,0.0998,5.2531,0f000001,0*2dd59142\n\t", "INSPVAXA,USB3,0,52.0,FINESTEERING,2107,283986.000,02000000,471d,15824;INS_ALIGNMENT_COMPLETE,INS_RTKFIXED,37.37030579801,126.72100988006,9.6428,22.3000,-0.3555,-0.3000,0.0366,-1.295250272,1.014100957,214.138979775,0.4311,0.3032,0.5948,0.1121,0.0935,0.0806,0.0960,0.0999,5.2589,0f000001,0*23ad1ff8\n\t", "INSPVAXA,USB3,0,52.0,FINESTEERING,2107,283987.000,02000000,471d,15824;INS_ALIGNMENT_COMPLETE,INS_RTKFIXED,37.37030239327,126.72100663816,9.6587,22.3000,-0.3682,-0.2898,0.0587,-1.329893089,1.153647504,213.823414970,0.4310,0.3029,0.5945,0.1121,0.0935,0.0803,0.0960,0.0999,5.2604,0f000001,0*f674c8ef\n\t", "INSPVAXA,USB3,0,49.5,FINESTEERING,2107,283987.500,02000000,471d,15824;INS_ALIGNMENT_COMPLETE,INS_RTKFIXED,37.37030066241,126.72100502191,9.6668,22.3000,-0.3610,-0.3081,0.0180,-1.422130124,0.889324413,213.618378707,0.4310,0.3029,0.5940,0.1122,0.0936,0.0801,0.0959,0.0999,5.2619,0f000001,0*76fbb7ae\n\t", "INSPVAXA,USB3,0,49.5,FINESTEERING,2107,283988.000,02000000,471d,15824;INS_ALIGNMENT_COMPLETE,INS_RTKFIXED,37.37029896329,126.72100339526,9.6748,22.3000,-0.3691,-0.2999,0.0388,-1.192200282,0.602579891,213.591513237,0.4310,0.3029,0.5940,0.1122,0.0936,0.0801,0.0959,0.0999,5.2619,0f000001,0*354c1358\n\t", "INSPVAXA,USB3,0,48.5,FINESTEERING,2107,283989.500,02000000,471d,15824;INS_ALIGNMENT_COMPLETE,INS_RTKFIXED,37.37029378078,126.72099856141,9.6916,22.3000,-0.3611,-0.2878,0.0332,-0.977406801,0.664431366,213.036331796,
